vi "Read UUT Data.vi"(8 "error in (no error)":errorcluster, 10 "Number Bytes To Read (256)":i32=256, 11 "VISA resource name":refnum<visa-resource-name>) -> (0 "error out":errorcluster, 1 "UUT Data":string, 2 "NumBytes Read":i32, 3 "VISA resource name out":refnum<visa-resource-name>)   [LabVIEW 2013, in "Fluke 5XXX Series Multicalibrators.lvlib"]
doc: "This VI returns data from the UUT in IEEE-488.2 Standard format over the Calibrator rear panel SERIAL 2 TO UUT serial port. The command may be sent over gpib or RS-232 ports, but applies to SERIAL 2 TO UUT serial port operation.\n\nNote:\n\nThis VI is available only for instrument models 5500A and 5520A."
uses:
  Fluke 5XXX Series Multicalibrators.lvlib
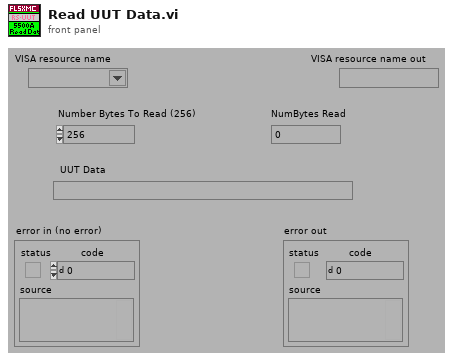
[diagram p1: front panel]
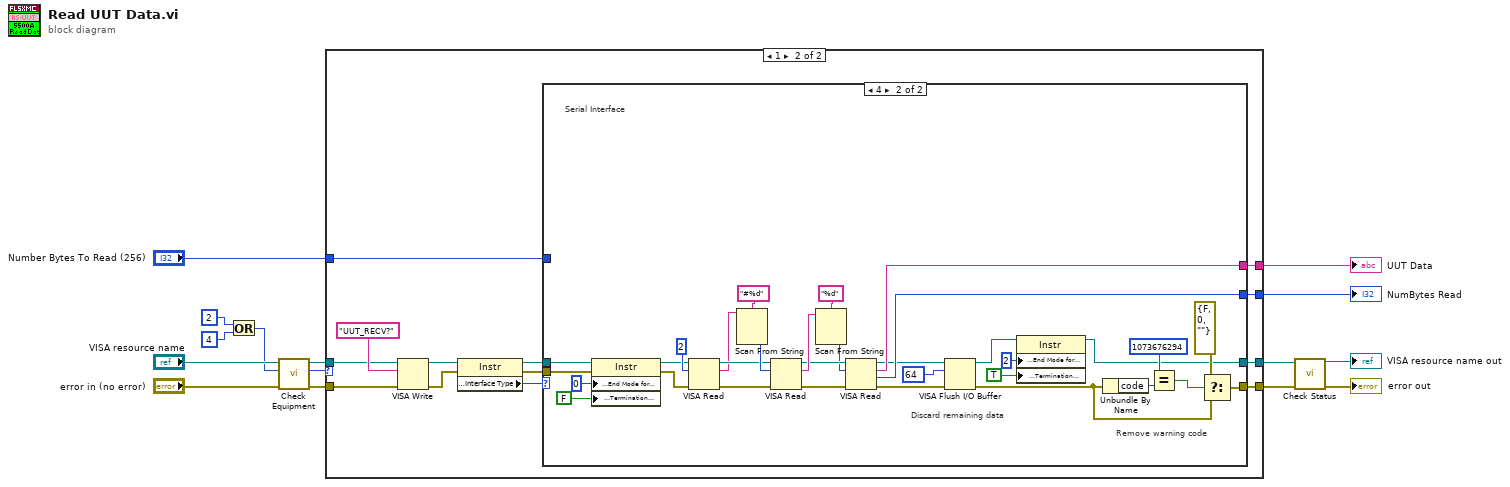
[diagram p0: block diagram]
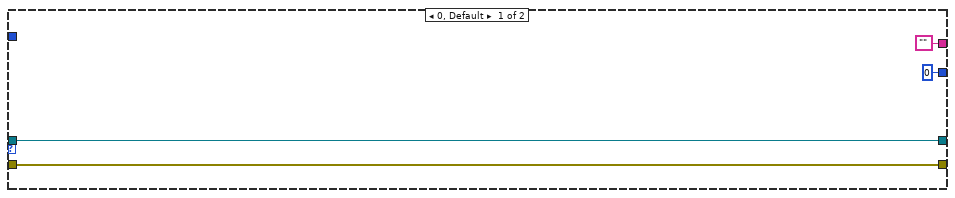
[diagram p2: hidden frame]
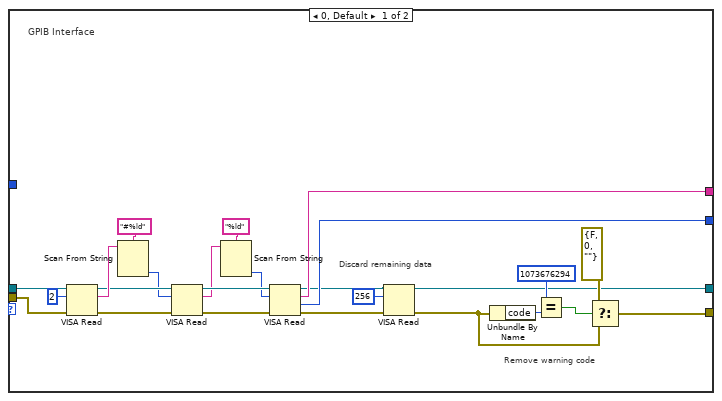
[diagram p3: hidden frame]
diagram:
  n1 = Or(x=u32 2, y=u32 4) -> (x .or. y?=w11:u32)
  n2 = call "Check Equipment.vi"("error in (no error)"="error in (no error)", "Bit Mask"=w11, "VISA resource name"="VISA resource name") -> ("error out"=w15:errorcluster, "Present?"=w8:u32, "VISA resource name out"=w14:refnum<visa-resource-name>)  [unwired: 6 in]
  n3 = case shown="1" w8 {
    tunnel: w15 -> [w18 w29]
    tunnel: w14 -> [w19 w28]
    tunnel: [w19 w23] -> w4
    tunnel: [w18 w22] -> w2
    tunnel: "Number Bytes To Read (256)" -> [_ w24]
    tunnel: ["" w21] -> w6
    tunnel: [u32 0 ("return count") w20] -> w5
    frame 0, Default {
    }
    frame 1 {
      n4 = VISA Write(VISA resource name=w28, write buffer="UUT_RECV?" ("write buffer (\"\")"), error in (no error)=w29) -> (VISA resource name out=w31:refnum<visa-resource-name>, error out=w30:errorcluster)  [unwired: 1 out]
      n5 = property class="Instr"(reference=w31, error in=w30) -> (reference out=w26:refnum<visa-resource-name>, error out=w25:errorcluster, "Interface Information:Interface Type"=w27:u16)
      n6 = case shown="4" w27 {
        tunnel: w26 -> [w57 w69]
        tunnel: w25 -> [w56 w68]
        tunnel: w24 -> [_ _]
        tunnel: [w35 w67] -> w23
        tunnel: [w40 w66] -> w22
        tunnel: [w52 w64] -> w21
        tunnel: [w38 w65] -> w20
        frame 0, Default {
          # "Discard remaining data"
          # "Remove warning code"
          # "GPIB Interface"
          n7 = VISA Read(VISA resource name=w57, byte count=u32 2 ("byte count (0)"), error in (no error)=w56) -> (VISA resource name out=w49:refnum<visa-resource-name>, read buffer=w53:string, error out=w51:errorcluster)  [unwired: 1 out]
          n8 = Scan From String(format string="#%ld", input string=w53) -> (output 1=w45:i32)  [unwired: 3 in, 3 out]
          n9 = VISA Read(VISA resource name=w49, byte count=w45, error in (no error)=w51) -> (VISA resource name out=w47:refnum<visa-resource-name>, read buffer=w46:string, error out=w50:errorcluster)  [unwired: 1 out]
          n10 = Scan From String(format string="%ld", input string=w46) -> (output 1=w39:i32)  [unwired: 3 in, 3 out]
          n11 = VISA Read(VISA resource name=w47, byte count=w39, error in (no error)=w50) -> (VISA resource name out=w36:refnum<visa-resource-name>, read buffer=w52:string, return count=w38:u32, error out=w37:errorcluster)
          n12 = VISA Read(VISA resource name=w36, byte count=u32 256 ("byte count (0)"), error in (no error)=w37) -> (VISA resource name out=w35:refnum<visa-resource-name>, error out=w34:errorcluster)  [unwired: 2 out]
          n13 = Unbundle By Name(w34) -> ("code"=w41:i32)
          n14 = Equal?(x=1073676294, y=w41) -> (x = y?=w43:bool)
          n15 = Select(t=errorcluster {"status"=FALSE, "code"=0, "source"=""} ("error out"), s=w43, f=w34) -> (s? t:f=w40:errorcluster)
        }
        frame 4 {
          # "Discard remaining data"
          # "Remove warning code"
          # "Serial Interface"
          n16 = property class="Instr"(reference=w69, error in=w68, "Serial Settings:End Mode for Reads"=u16 0 ("ASRL End In"), "Message Based Settings:Termination Character Enable"=FALSE ("TermChar En")) -> (reference out=w76:refnum<visa-resource-name>, error out=w77:errorcluster)
          n17 = VISA Read(VISA resource name=w76, byte count=u32 2 ("byte count (0)"), error in (no error)=w77) -> (VISA resource name out=w81:refnum<visa-resource-name>, read buffer=w80:string, error out=w82:errorcluster)  [unwired: 1 out]
          n18 = Scan From String(format string="#%d", input string=w80) -> (output 1=w83:i32)  [unwired: 3 in, 3 out]
          n19 = VISA Read(VISA resource name=w81, byte count=w83, error in (no error)=w82) -> (VISA resource name out=w72:refnum<visa-resource-name>, read buffer=w84:string, error out=w73:errorcluster)  [unwired: 1 out]
          n20 = Scan From String(format string="%d", input string=w84) -> (output 1=w63:i32)  [unwired: 3 in, 3 out]
          n21 = VISA Read(VISA resource name=w72, byte count=w63, error in (no error)=w73) -> (VISA resource name out=w62:refnum<visa-resource-name>, read buffer=w64:string, return count=w65:u32, error out=w61:errorcluster)
          n22 = VISA Flush I/O Buffer(VISA resource name=w62, mask (16)=u32 64, error in (no error)=w61) -> (VISA resource name out=w59:refnum<visa-resource-name>, error out=w60:errorcluster)
          n23 = property class="Instr"(reference=w59, "Serial Settings:End Mode for Reads"=u16 2 ("ASRL End In"), "Message Based Settings:Termination Character Enable"=TRUE ("TermChar En")) -> (reference out=w67:refnum<visa-resource-name>)  [unwired: 1 in, 1 out]
          n24 = Unbundle By Name(w60) -> ("code"=w86:i32)
          n25 = Equal?(x=1073676294, y=w86) -> (x = y?=w88:bool)
          n26 = Select(t=errorcluster {"status"=FALSE, "code"=0, "source"=""} ("error out"), s=w88, f=w60) -> (s? t:f=w66:errorcluster)
        }
      }
    }
  }
  "UUT Data" <- w6
  "NumBytes Read" <- w5
  n27 = call "Check Status.vi"("VISA resource name"=w4, "error in (no error)"=w2) -> ("VISA resource name out"=→"VISA resource name out":refnum<visa-resource-name>, "error out"=→"error out":errorcluster)  [unwired: 12 in]
